vi "Write.vi"(8 "error in (no error)":errorcluster, 9 "Variant":variant, 10 "String":string, 11 "AK TCP in":refnum<class "AK TCP.lvclass">) -> (0 "error out":errorcluster, 3 "AK TCP out":refnum<class "AK TCP.lvclass">)   [LabVIEW 2023, in "Protocols.lvlib" / "AK TCP.lvclass"]
uses:
  AK TCP.lvclass
  TCP/TCP.lvclass
  Protocols.lvlib
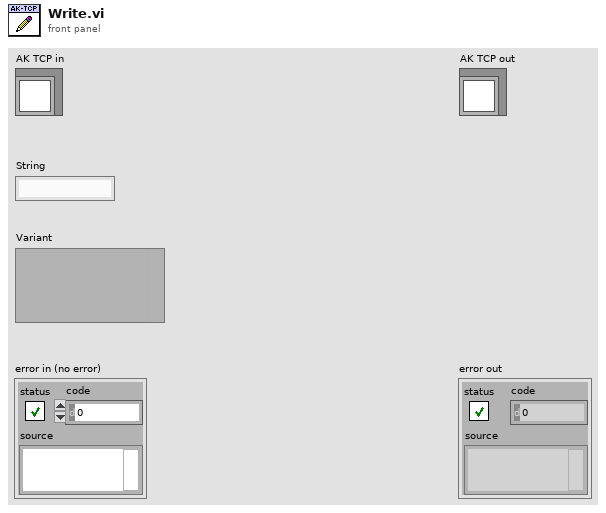
[diagram p1: front panel]
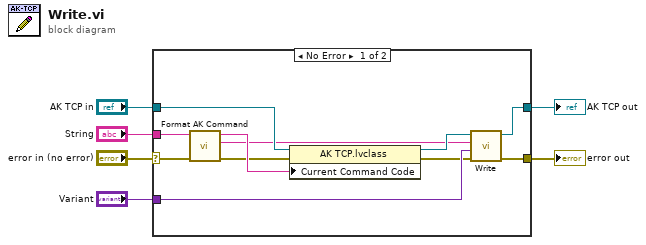
[diagram p0: block diagram]
diagram:
  n1 = case shown="No Error" "error in (no error)" {
    selector: "error in (no error)" -> [w11 w19]
    tunnel: [w17 w19] -> w2
    tunnel: [w16 w18] -> w1
    tunnel: "Variant" -> [w8 _]
    tunnel: "String" -> [w15 _]
    tunnel: "AK TCP in" -> [w14 w18]
    frame No Error {
      n2 = call "Format AK Command.vi"("error in (no error)"=w11, "String in"=w15) -> ("error out"=w12:errorcluster, "Command"=w9:string, "Command Code"=w13:string)  [unwired: 7 in]
      n3 = property class="AK TCP.lvclass"(reference=w14, error in=w12, "Current Command Code"=w13) -> (reference out=w10:refnum<class "AK TCP.lvclass">, error out=w7:errorcluster)
      n4 = call-parent "Write.vi"("error in (no error)"=w7, "Variant"=w8, "String"=w9, "Ethernet in"=w10) -> ("error out"=w17:errorcluster, "Ethernet out"=w16:refnum<class "AK TCP.lvclass">)  [unwired: 6 in]
    }
    frame Error {
    }
  }
  "error out" <- w2
  "AK TCP out" <- w1
